vi "eLog.vi"(3 "error in":errorcluster, 4 "Device ID":string, 5 "fileRefIn":refnum<file>) -> (0 "error out":errorcluster, 2 "This VI":refnum<vi>)   [LabVIEW 2012]
doc: "<B>Handle Exceptions</B> handles all errors generated at run time. Any errors generated are first queued up and sent to the main VI where they may viewed by the user, then written to an erro log and finally cleared so as to prevent communication failures. The icon design is courtesy of Justin Langridge."
panel:
  in  "# to Write":i32=20
  out "Error Log":string[][](table)
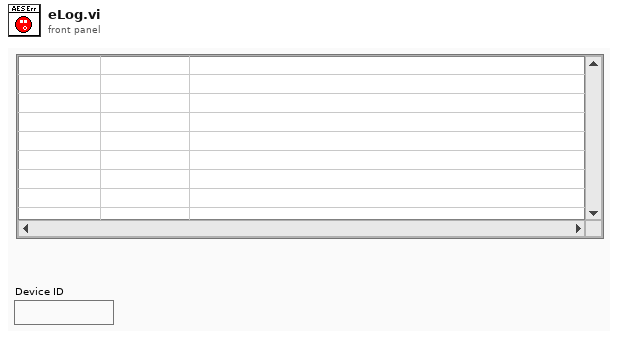
[diagram p1: front panel]
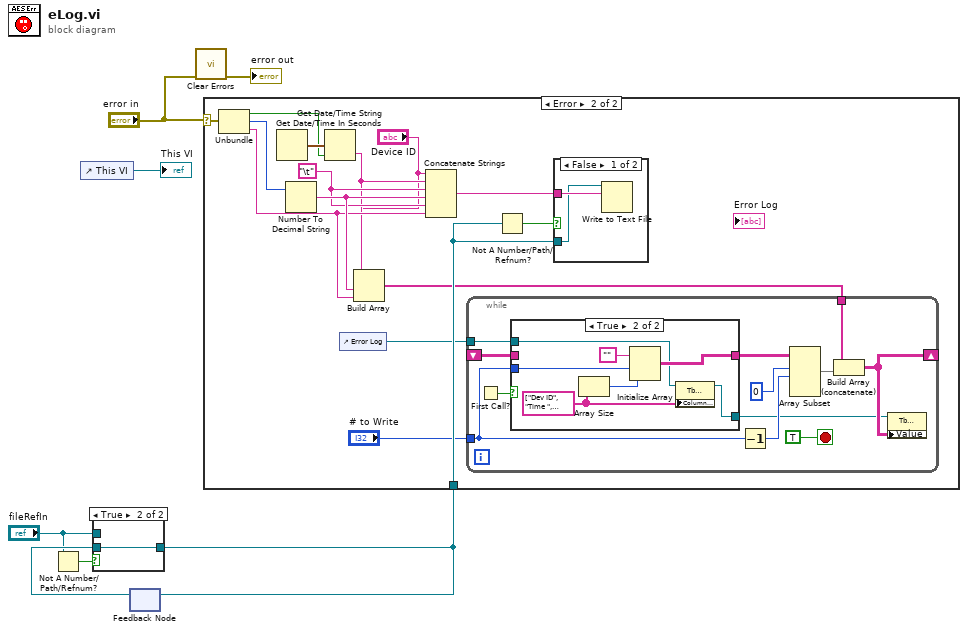
[diagram p0: block diagram]
diagram:
  n1 = Not A Number/Path/Refnum?(number/path/refnum="fileRefIn") -> (NaN/Path/Refnum?=w7:bool)
  n2 = control-ref of="This VI"() -> (→"This VI":refnum<vi>)
  n3 = feedback #1() -> (w2:refnum<file>)  [unwired: 1 in]
  n4 = case shown="True" w7 {
    tunnel: "fileRefIn" -> [w8 _]
    tunnel: [w8 w9] -> w3
    tunnel: w2 -> [_ w9]
    frame False {
    }
    frame True {
    }
  }
  n5 = feedback-in #1(w3) -> ()
  n6 = call <vilib>:"Clear Errors.vi"("error in (no error)"="error in") -> ("error out"=→"error out":errorcluster)  [unwired: 6 out]
  n7 = case shown="Error" "error in" {
    selector: "error in" -> [_ w24]
    tunnel: w3 -> [_ w14]
    frame No Error {
    }
    frame Error {
      w21 = "\t"
      n8 = Unbundle(w24) -> ("status"=w17:bool, "code"=w22:i32, "source"=w19:string)
      n9 = Get Date/Time In Seconds() -> (seconds since 1Jan1904=w20:timestamp)
      n10 = Number To Decimal String(number=w22) -> (decimal integer string=w23:string)  [unwired: 1 out]
      n11 = Get Date/Time String(seconds (now)=w20, want seconds? (F)=w17) -> (time string=w18:string)  [unwired: 2 out]
      n12 = control-ref of="Error Log"() -> (w13:refnum<vi>)
      n13 = Build Array("Device ID", w18, w23, w19) -> (w11:string[])
      n14 = Concatenate Strings("Device ID", w18, w21, w23, w21, w19) -> (w15:string)
      n15 = while {
        shift-right: [w32] -> _
        shift-left: _ -> [w31]
        tunnel: w13 -> [w26]
        tunnel: "# to Write" -> [w28]
        tunnel: w11 -> [w27]
        stop <- TRUE ("stop") stop-if-true
        n16 = First Call?() -> (First Call?: T/F=w29:bool)
        n17 = case shown="True" w29 {
          tunnel: [w38 w44] -> w30
          tunnel: w28 -> [_ w43]
          tunnel: w31 -> [w38 _]
          tunnel: w26 -> [w37 w42]
          tunnel: [w37 w41] -> w25
          frame False {
          }
          frame True {
            w40 = string[] ["Dev ID", "Time ", "Error Code", "Error Message"] ("Column Header Strings[]")
            n18 = Array Size(array=w40) -> (size(s)=w39:i32)
            n19 = Initialize Array("", w43, w39) -> (w44:string[][])
            n20 = property class="Tbl (strict)"(reference=w42, "Column Headers[]"=w40) -> (reference out=w41:refnum<vi>)  [unwired: 1 in, 1 out]
          }
        }
        n21 = Decrement(x=w28) -> (x-1=w35:i32)
        n22 = Array Subset(array=w30, index (row)=0 ("index"), length (row)=w35) -> (w34:string[][])  [unwired: 2 in]
        n23 = Build Array (concatenate)(w27, w34) -> (w32:string[][])
        n24 = property class="Tbl (strict)"(reference=w25, "Value"=w32) -> ()  [unwired: 1 in, 2 out]
      }
      n25 = Not A Number/Path/Refnum?(number/path/refnum=w14) -> (NaN/Path/Refnum?=w16:bool)
      n26 = case shown="False" w16 {
        tunnel: w15 -> [w47 _]
        tunnel: w14 -> [w46 _]
        frame False {
          n27 = Write to Text File(file (use dialog)=w46, text=w47) -> ()  [unwired: 2 in, 3 out]
        }
        frame True {
        }
      }
    }
  }
